vi "Globals.vi"() -> ()   [LabVIEW 2019]
panel:
  in  "SA deaths URL":string="https://raw.githubusercontent.com/dsfsi/covid19za/master/data/covid19za_provincial_cumulative_timeline_deaths.csv"
  in  "SA cases URL":string="https://raw.githubusercontent.com/dsfsi/covid19za/master/data/covid19za_provincial_cumulative_timeline_confirmed.csv"
  in  "US cases URL":string="https://raw.githubusercontent.com/CSSEGISandData/COVID-19/master/csse_covid_19_data/csse_covid_19_time_series/time_series_covid19_confirmed_US.csv"
  in  "US deaths URL":string="https://raw.githubusercontent.com/CSSEGISandData/COVID-19/master/csse_covid_19_data/csse_covid_19_time_series/time_series_covid19_deaths_US.csv"
  in  "Global populations URL":string="https://raw.githubusercontent.com/CSSEGISandData/COVID-19/master/csse_covid_19_data/UID_ISO_FIPS_LookUp_Table.csv"
  in  "Global cases URL":string="https://raw.githubusercontent.com/CSSEGISandData/COVID-19/master/csse_covid_19_data/csse_covid_19_time_series/time_series_covid19_confirmed_global.csv"
  in  "Global deaths URL":string="https://raw.githubusercontent.com/CSSEGISandData/COVID-19/master/csse_covid_19_data/csse_covid_19_time_series/time_series_covid19_deaths_global.csv"
  in  "version":u32=33
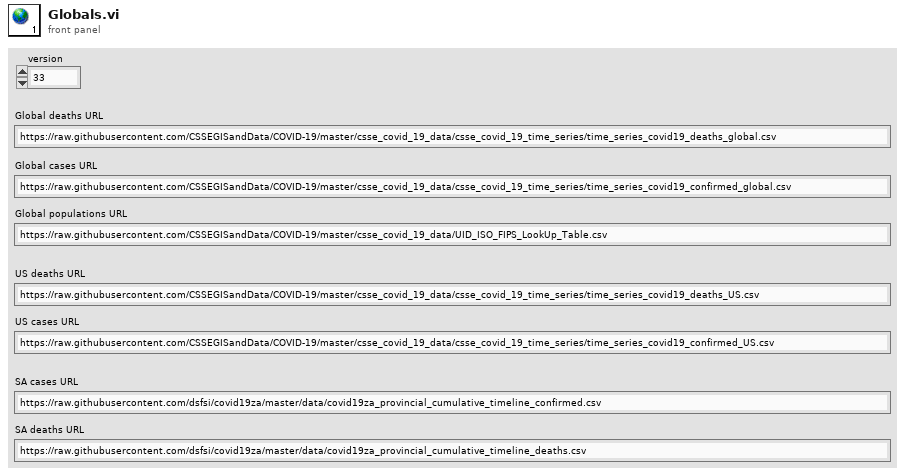
[diagram p1: front panel]
diagram:
